vi "SetTempSetpointParam.vi"(8 "error in (no error)":errorcluster, 10 "TSetpoint(degC/100)":i16, 11 "hcam in":i16) -> (0 "error out":errorcluster, 1 "Success":bool, 2 "TSetpointReadback(degC/100)":i16, 3 "hcam out":i16)   [LabVIEW 2013]
uses:
  PARAM_ID_TypDef.ctl
  SetParamCurrentValue(I16).vi
  GetParameterValue(I16).vi
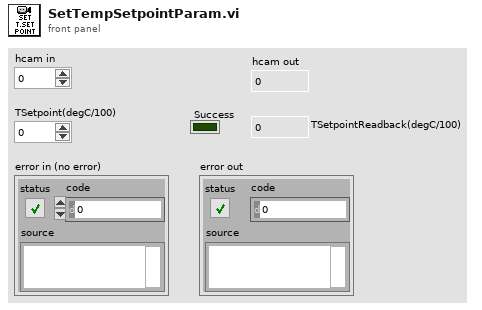
[diagram p1: front panel]
types:
  T1 = typedef "PARAM_ID_TypDef.ctl" = u32
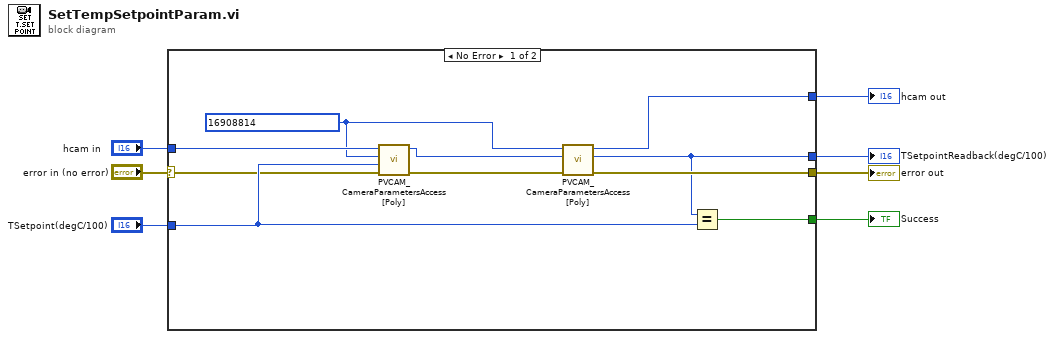
[diagram p0: block diagram]
diagram:
  n1 = case shown="No Error" "error in (no error)" {
    selector: "error in (no error)" -> [w8 w19]
    tunnel: [w17 _] -> w7
    tunnel: "TSetpoint(degC/100)" -> [w16 _]
    tunnel: [w15 w19] -> w5
    tunnel: "hcam in" -> [w13 w18]
    tunnel: [w10 _] -> w3
    tunnel: [w9 w18] -> w2
    frame No Error {
      w11 = T1 16908814 ("Param ID (Ring)")
      n2 = call-poly "PVCAM_CameraParametersAccess[Poly].vi"("error in (no error)"=w8, "param_value"=w16, "Param ID (Ring)"=w11, "hcam in"=w13) -> ("error out"=w12:errorcluster, "hcam out"=w14:i16)  [unwired: 5 in, 1 out]
      n3 = call-poly "PVCAM_CameraParametersAccess[Poly].vi"("error in (no error)"=w12, "hcam in"=w14, "Param ID (Ring)"=w11) -> ("error out"=w15:errorcluster, "ParameterValue"=w10:i16, "hcam out"=w9:i16)  [unwired: 6 in]
      n4 = Equal?(x=w10, y=w16) -> (x = y?=w17:bool)
    }
    frame Error {
    }
  }
  "Success" <- w7
  "TSetpointReadback(degC/100)" <- w3
  "error out" <- w5
  "hcam out" <- w2
